vi "MEM IO Write__ogtk.vi"   [LabVIEW 2020]
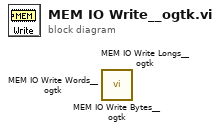
[diagram p0: block diagram]
diagram:
  n1 = call <userlib>:"MEM IO Write Bytes__ogtk.vi"() -> ()  [unwired: 7 in, 1 out]
  n2 = call <userlib>:"MEM IO Write Longs__ogtk.vi"() -> ()  [unwired: 7 in, 1 out]
  n3 = call <userlib>:"MEM IO Write Words__ogtk.vi"() -> ()  [unwired: 7 in, 1 out]
